vi "Gyro-adjusted-arcade.vi"(7 "Rotate deadband":dbl=0.1 format="%#_13g", 8 "gyro in (deg)":dbl, 9 "Right X in":dbl, 10 "Left X in":dbl, 11 "Y in":dbl) -> (0 "Right out":dbl, 3 "Left out":dbl)   [LabVIEW 2016]
uses:
  <vilib>/Analysis/coordinate.llb/2D Cartesian Coordinate Rotation (Scalar).vi
  <vilib>/Analysis/NI_AALPro.lvlib
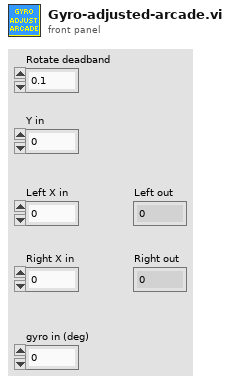
[diagram p1: front panel]
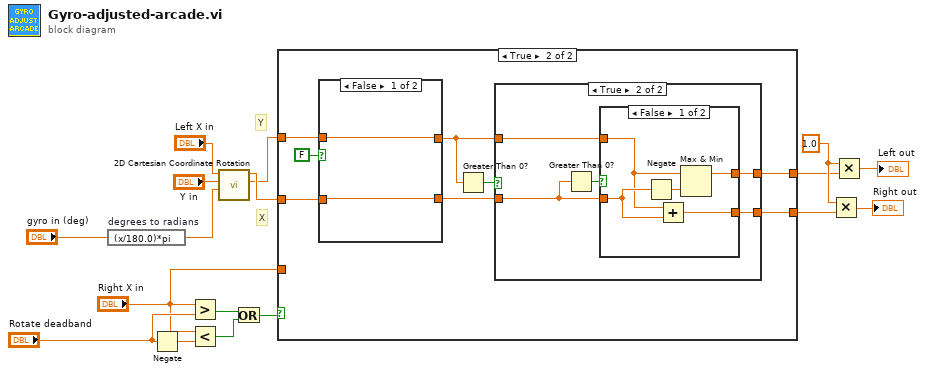
[diagram p0: block diagram]
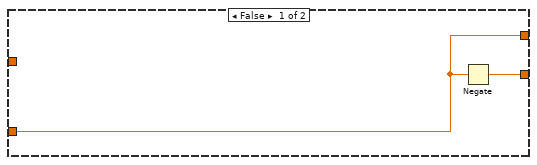
[diagram p2: hidden frame]
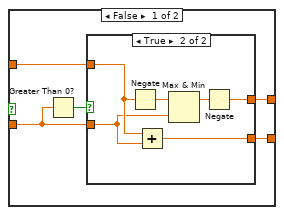
[diagram p3: hidden frame]
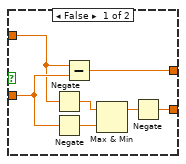
[diagram p4: hidden frame]
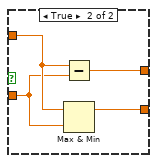
[diagram p5: hidden frame]
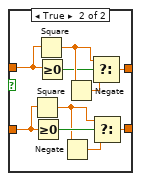
[diagram p6: hidden frame]
diagram:
  w5 = 1.0 ("Max Output")
  # "X"
  # "Y"
  n1 = expression code="(x/180.0)*pi" "degrees to radians"("gyro in (deg)") -> (w14:dbl)
  n2 = Negate(x="Rotate deadband") -> (-x=w8:dbl)
  n3 = Greater?(x="Right X in", y="Rotate deadband") -> (0:w10:bool)
  n4 = Less?(x="Right X in", y=w8) -> (x < y?=w9:bool)
  n5 = call-poly <vilib>:"2D Cartesian Coordinate Rotation.vi"("theta"=w14, "y"="Y in", "x"="Left X in") -> ("y out"=w12:dbl, "x out"=w13:dbl)  [unwired: 6 in, 1 out]
  n6 = Or(x=w10, y=w9) -> (x .or. y?=w11:bool)
  n7 = case shown="True" w11 {
    tunnel: w13 -> [_ w23]
    tunnel: w12 -> [_ w22]
    tunnel: "Right X in" -> [w18 _]
    tunnel: [w18 w21] -> w4
    tunnel: [w19 w20] -> w3
    frame False {
      n8 = Negate(x=w18) -> (-x=w19:dbl)
    }
    frame True {
      n9 = case shown="False" FALSE ("Square Inputs") {
        tunnel: [w60 w71] -> w25
        tunnel: [w61 w70] -> w26
        tunnel: w23 -> [w60 w69]
        tunnel: w22 -> [w61 w68]
        frame False {
        }
        frame True {
          n10 = Square(x=w69) -> (x^2=w66:dbl)
          n11 = Greater Or Equal To 0?(x=w69) -> (x >= 0?=w67:bool)
          n12 = Square(x=w68) -> (x^2=w63:dbl)
          n13 = Greater Or Equal To 0?(x=w68) -> (x >= 0?=w62:bool)
          n14 = Negate(x=w66) -> (-x=w65:dbl)
          n15 = Negate(x=w63) -> (-x=w64:dbl)
          n16 = Select(t=w63, s=w62, f=w64) -> (s? t:f=w70:dbl)
          n17 = Select(t=w66, s=w67, f=w65) -> (s? t:f=w71:dbl)
        }
      }
      n18 = Greater Than 0?(x=w26) -> (x > 0?=w27:bool)
      n19 = case shown="True" w27 {
        tunnel: w25 -> [w31 w49]
        tunnel: w26 -> [w30 w48]
        tunnel: [w29 w47] -> w21
        tunnel: [w28 w46] -> w20
        frame False {
          n20 = Greater Than 0?(x=w31) -> (x > 0?=w32:bool)
          n21 = case shown="True" w32 {
            tunnel: w31 -> [w39 w41]
            tunnel: w30 -> [w37 w42]
            tunnel: [w33 w43] -> w29
            tunnel: [w34 w40] -> w28
            frame False {
              n22 = Negate(x=w37) -> (-x=w38:dbl)
              n23 = Negate(x=w39) -> (-x=w36:dbl)
              n24 = Subtract(x=w37, y=w39) -> (x-y=w33:dbl)
              n25 = Max & Min(x=w38, y=w36) -> (max(x,y)=w35:dbl)  [unwired: 1 out]
              n26 = Negate(x=w35) -> (-x=w34:dbl)
            }
            frame True {
              n27 = Negate(x=w42) -> (-x=w45:dbl)
              n28 = Add(x=w42, y=w41) -> (x+y=w40:dbl)
              n29 = Max & Min(x=w45, y=w41) -> (max(x,y)=w44:dbl)  [unwired: 1 out]
              n30 = Negate(x=w44) -> (-x=w43:dbl)
            }
          }
        }
        frame True {
          n31 = Greater Than 0?(x=w49) -> (x > 0?=w50:bool)
          n32 = case shown="False" w50 {
            tunnel: w49 -> [w55 w57]
            tunnel: w48 -> [w52 w58]
            tunnel: [w53 w56] -> w47
            tunnel: [w51 w59] -> w46
            frame False {
              n33 = Negate(x=w55) -> (-x=w54:dbl)
              n34 = Add(x=w52, y=w55) -> (x+y=w51:dbl)
              n35 = Max & Min(x=w52, y=w54) -> (max(x,y)=w53:dbl)  [unwired: 1 out]
            }
            frame True {
              n36 = Subtract(x=w58, y=w57) -> (x-y=w56:dbl)
              n37 = Max & Min(x=w58, y=w57) -> (max(x,y)=w59:dbl)  [unwired: 1 out]
            }
          }
        }
      }
    }
  }
  n38 = Multiply(x=w5, y=w3) -> (x*y=→"Right out":dbl)
  n39 = Multiply(x=w5, y=w4) -> (x*y=→"Left out":dbl)
